vi "Termo_1.5__.vi"() -> ()   [LabVIEW 2015]
doc: "Программа мониторинга температуры"
panel:
  out "?":bool
  out "graph_update":bool
  out "Конфиг. АЦП?":bool
  in  "Tab Control":enum32{"ИЗМЕРЕНИЯ [К]", " АЦП", "ГРАФИК"}(tab)
  out "R2":dbl format="%.2f"
  in  "T2_visible":bool=TRUE
  in  "T5_visible":bool=TRUE
  out "R1":dbl format="%.2f"
  in  "T1_visible":bool=TRUE
  in  "T3_visible":bool=TRUE
  in  "T4_visible":bool=TRUE
  in  "T6_visible":bool=TRUE
  in  "stop":bool
  in  "ADC_dyn_range":T1(ring)=enum."± 0.625 В"
  in  "Buf_size":u8=1 min=1 max=128
  in  "SPS":T2(ring)
  in  "IP-адрес":string="192.168.127.254"
  in  "порт":u16=4001
  in  "Очистить график":bool
  in  "load_coeff.":bool caption="Disconn"
  in  "save_coeff.":bool caption="Disconn"
  in  "Coeff_cl_ch5":T3={"k1"=19.4736079181311652, "k2"=-232.79779903171584, "k3"=1229.13228608109057005, "k4"=-3103.0388431325554801, "k5"=4219.3520172238349901, "k6"=-2697.7160155214369299, "k7"=779.55193291697651198} caption="Канал 5" {"k7" format="%#_16g"; "k6" format="%#_16g"; "k5" format="%#_16g"; "k4" format="%#_16g"; "k3" format="%#_16g"; "k2" format="%#_16g"; "k1" format="%#_16g"}
  in  "Coeff_cl_ch4":T3={"k1"=24.218377729237545301, "k2"=-311.679773783311248, "k3"=1734.44359050504863, "k4"=-4665.87189712375402, "k5"=6719.3289510309696202, "k6"=-4578.02570509165525, "k7"=1400.00134176202118} caption="Канал 4" {"k7" format="%#_16g"; "k6" format="%#_16g"; "k5" format="%#_16g"; "k4" format="%#_16g"; "k3" format="%#_16g"; "k2" format="%#_16g"; "k1" format="%#_16g"}
  in  "Coeff_cl_ch3":T3={"k1"=8.756, "k2"=-142.210000000000000006, "k3"=1253.0, "k4"=-4877.1, "k5"=10581.0, "k6"=-10354.0, "k7"=3998.5} caption="Канал 3" {"k7" format="%#_16g"; "k6" format="%#_16g"; "k5" format="%#_16g"; "k4" format="%#_16g"; "k3" format="%#_16g"; "k2" format="%#_16g"; "k1" format="%#_16g"}
  in  "Coeff_cl_ch2":T3={"k1"=31.9101907935109921, "k2"=-399.867376562207937, "k3"=2119.32627579197288, "k4"=-5531.15447566658258, "k5"=7772.21873644739389, "k6"=-5292.23886113613844, "k7"=1613.2211984321475} caption="Канал 2" {"k7" format="%#_16g"; "k6" format="%#_16g"; "k5" format="%#_16g"; "k4" format="%#_16g"; "k3" format="%#_16g"; "k2" format="%#_16g"; "k1" format="%#_16g"}
  in  "Coeff_cl_ch6":T3={"k1"=11.9061392787261866, "k2"=-139.902402561856434, "k3"=774.882810204289854, "k4"=-1837.4832512177527, "k5"=2139.5822282396256899, "k6"=-730.555961686186492, "k7"=169.810834781266749} caption="Канал 6" {"k7" format="%#_16g"; "k6" format="%#_16g"; "k5" format="%#_16g"; "k4" format="%#_16g"; "k3" format="%#_16g"; "k2" format="%#_16g"; "k1" format="%#_16g"}
  in  "GraphLookB":bool
  in  "xScale -":bool
  in  "xScale +":bool
  out "мин.":string="1"
  in  "Старт измер.":bool
  in  "Стоп измер.":bool
  in  "Добавить время":dbl(ring)=300.0 items=["10 сек."=10.0, "1 мин."=60.0, "5 мин."=300.0, "20 мин."=1200.0]
  in  "min":dbl=4.0
  in  "max":dbl=300.0
  out "часы":string="0"
  in  "Autoscale":bool=TRUE
  out "сек.":string="0"
  out "Сутки":string
  out "счетчик":u32=4001
  in  "Запись в файл":bool
  in  "header?":bool caption="Disconn"
  out "con ID":refnum<k5>
  out "Graphs T":dynamicdata(graph) caption="U, мВ"
  # "U, мВ"
  # "Канал 1"
  # "Канал 2"
  # "Скорость измерений"
  # "SPS = Samples Per Second"
  # "Размер буфера усреднения"
  # "Диапазон измерений"
  # "Подключение"
  # "Шкала"
  # "Время графика"
  # ":"
  # ":"
  # "Измерения"
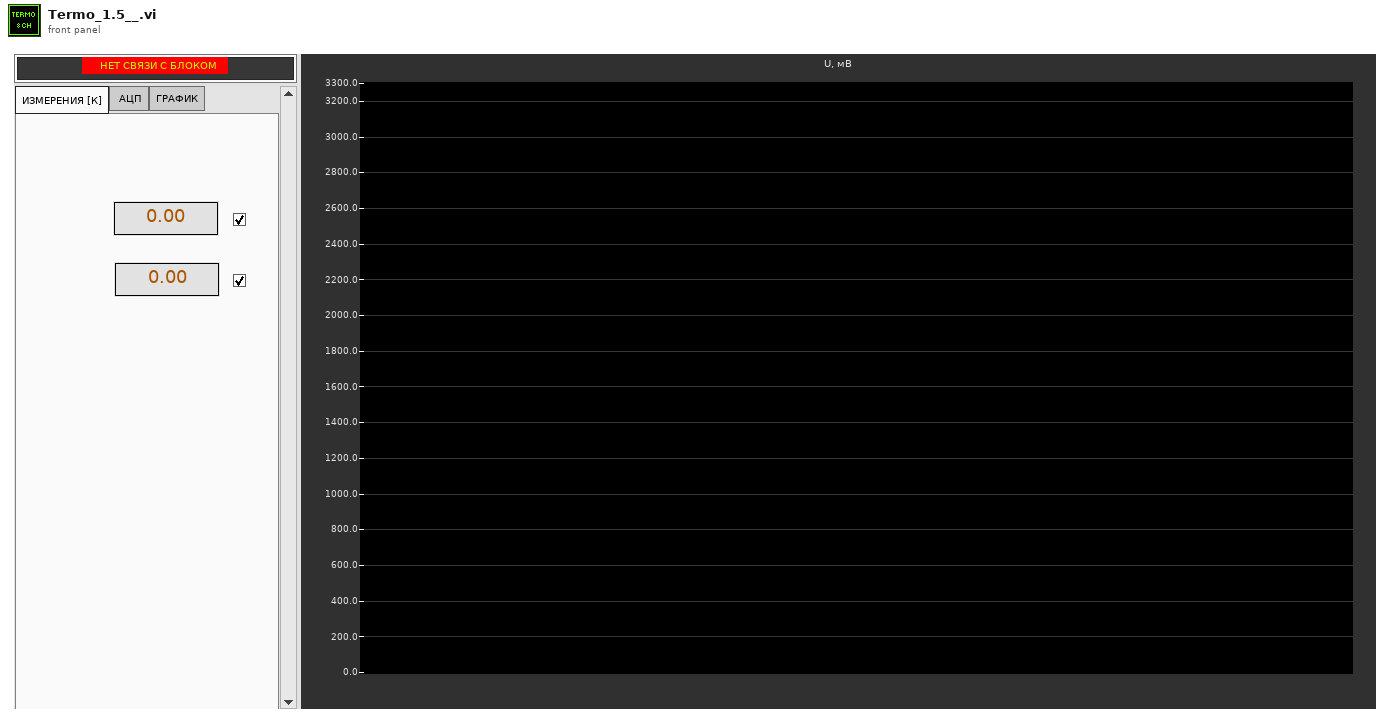
[diagram p1: front panel]
types:
  T1 = enum16{"± 5 В", "± 2.5 В", "± 1.25 В", "± 0.625 В", "± 312.5 мВ", "± 156.25 мВ", "± 78.125 мВ"}
  T2 = enum16{"2,5 SPS", "5 SPS", "10 SPS", "25 SPS", "50 SPS", "100 SPS", "500 SPS"}
  T3 = cluster{"k1":ext, "k2":ext, "k3":ext, "k4":ext, "k5":ext, "k6":ext, "k7":ext}
  T4 = enum32{"Page Enabled", "Page Disabled", "Page Disabled & Grayed"}
  T5 = enum16{"Standard", "Buffered", "CRLF", "Immediate"}
  T6 = typedef "LVDateTimeRec.ctl" = cluster{"fractional second":dbl, "second":i32, "minute":i32, "hour":i32, "day of month":i32, "month":i32, "year":i32, "day of week":i32, "day of year":i32, "DST":i32}
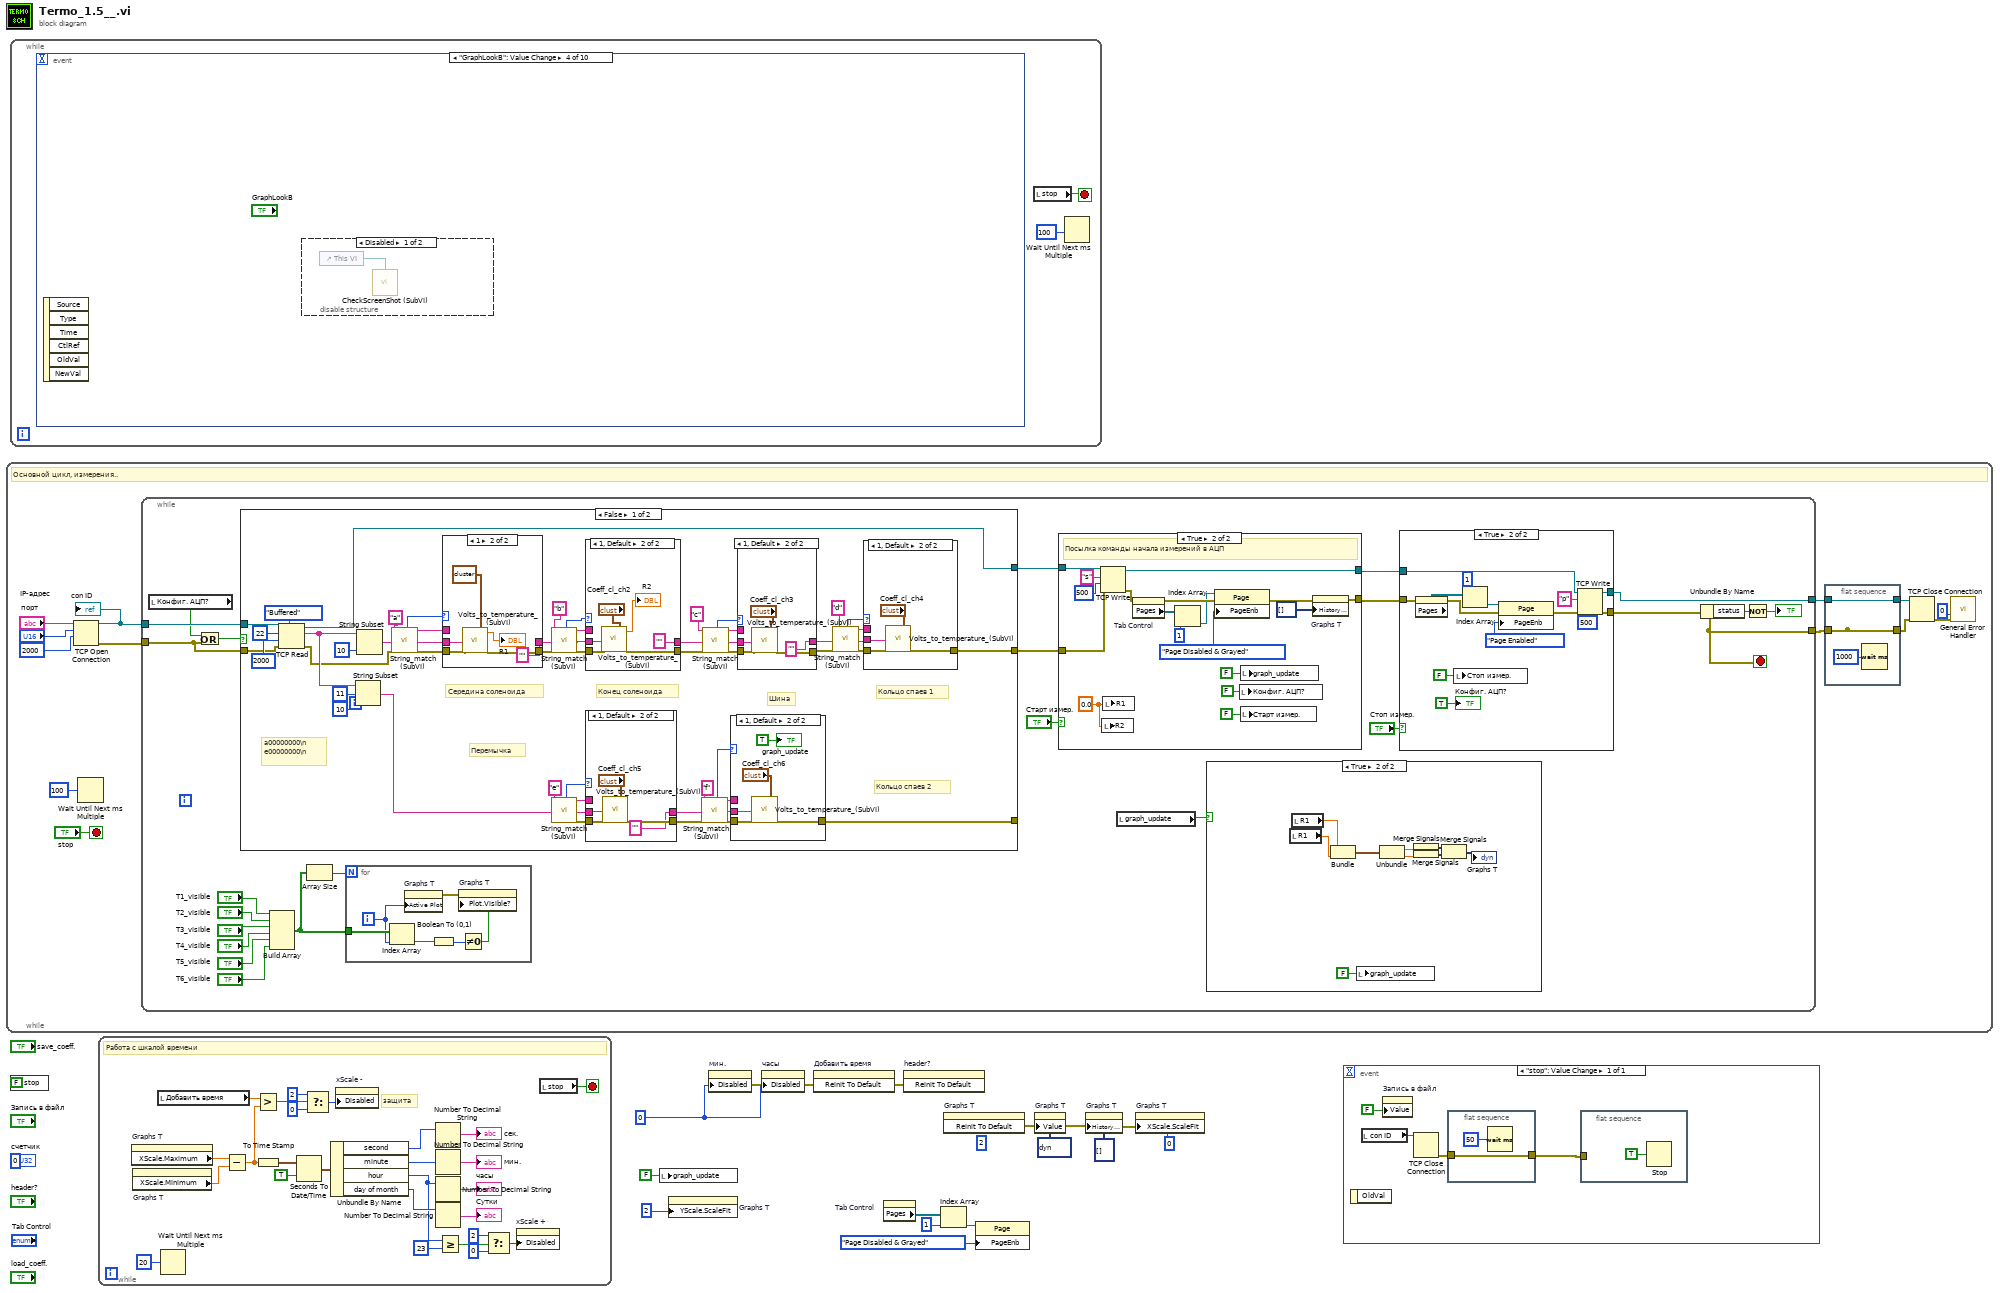
[diagram p0: block diagram]
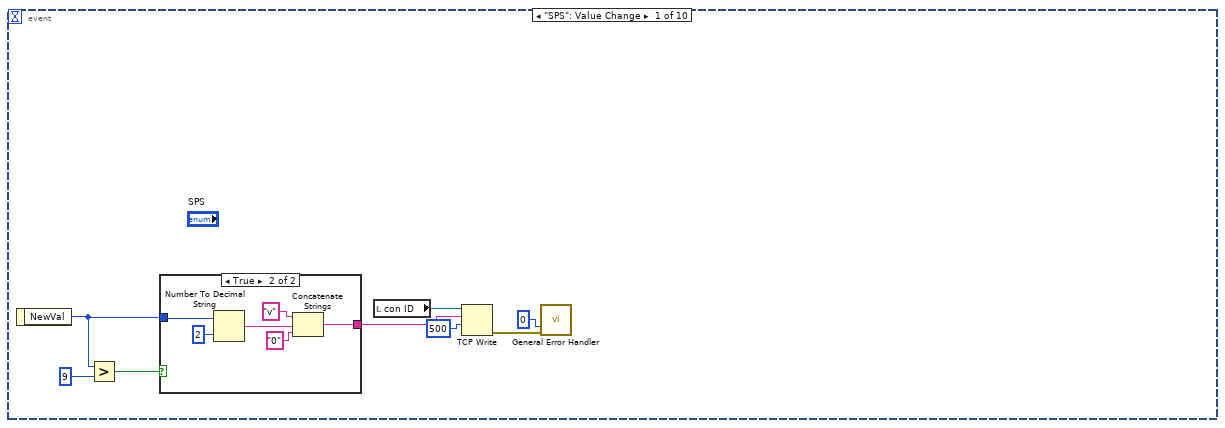
[diagram p2: hidden frame]
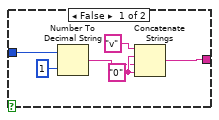
[diagram p3: hidden frame]
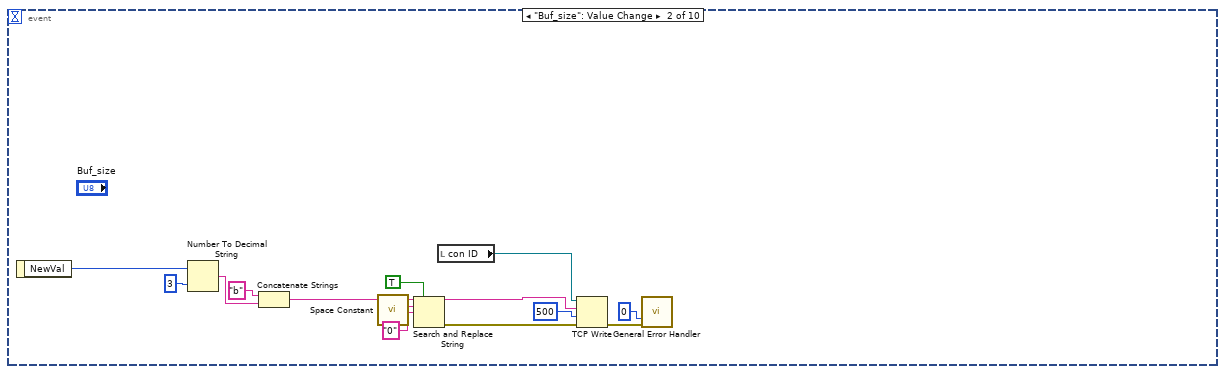
[diagram p4: hidden frame]
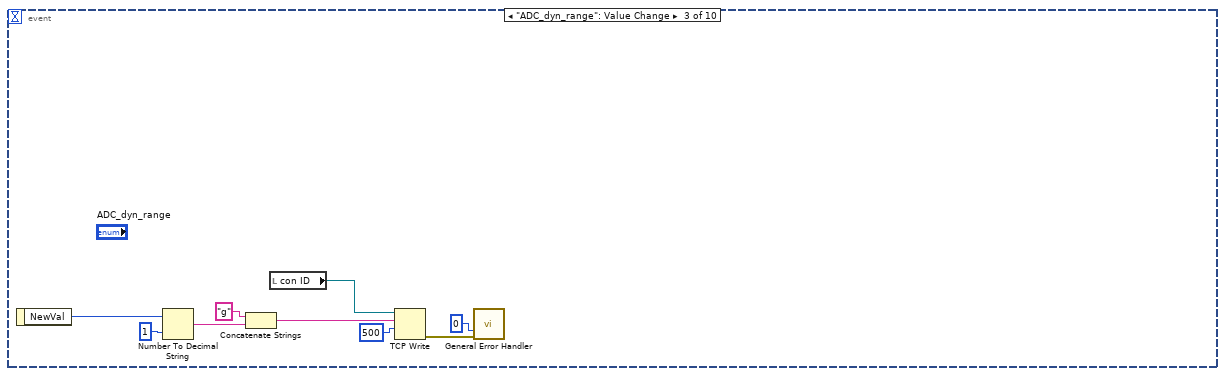
[diagram p5: hidden frame]
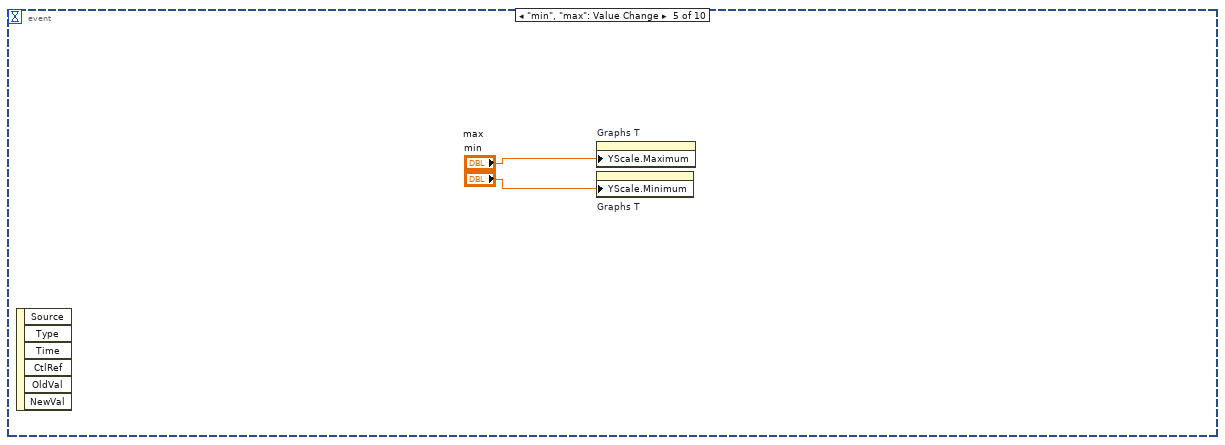
[diagram p7: hidden frame]
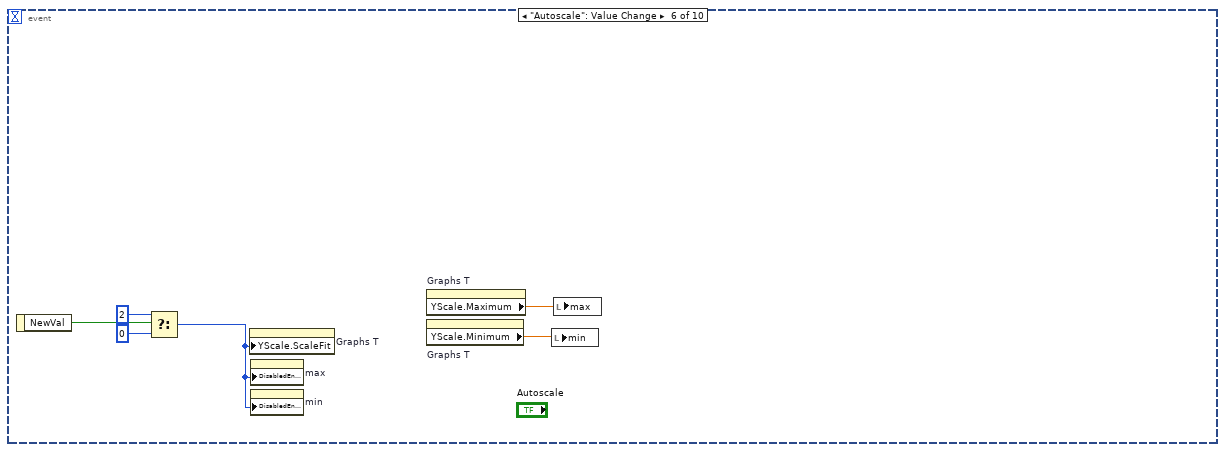
[diagram p8: hidden frame]
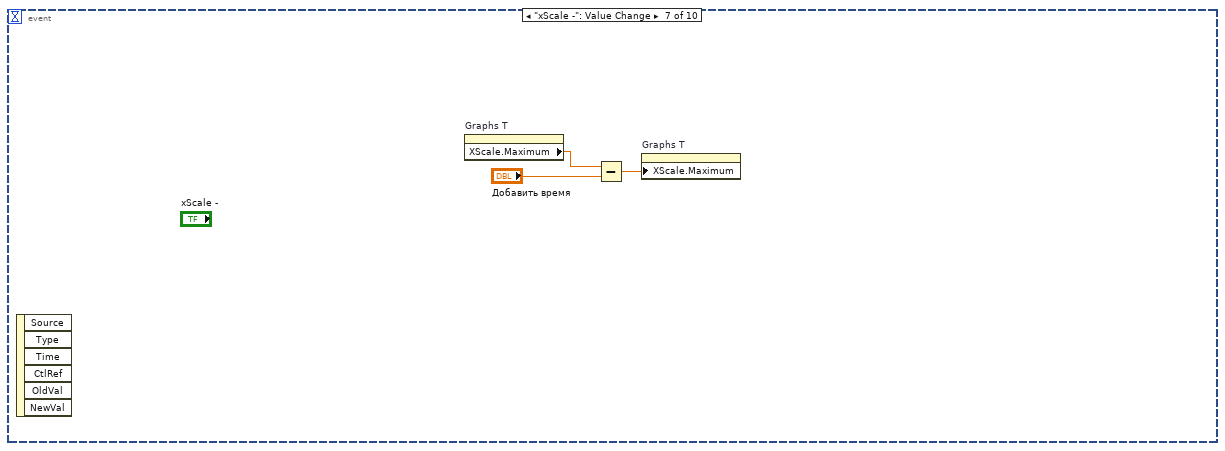
[diagram p9: hidden frame]
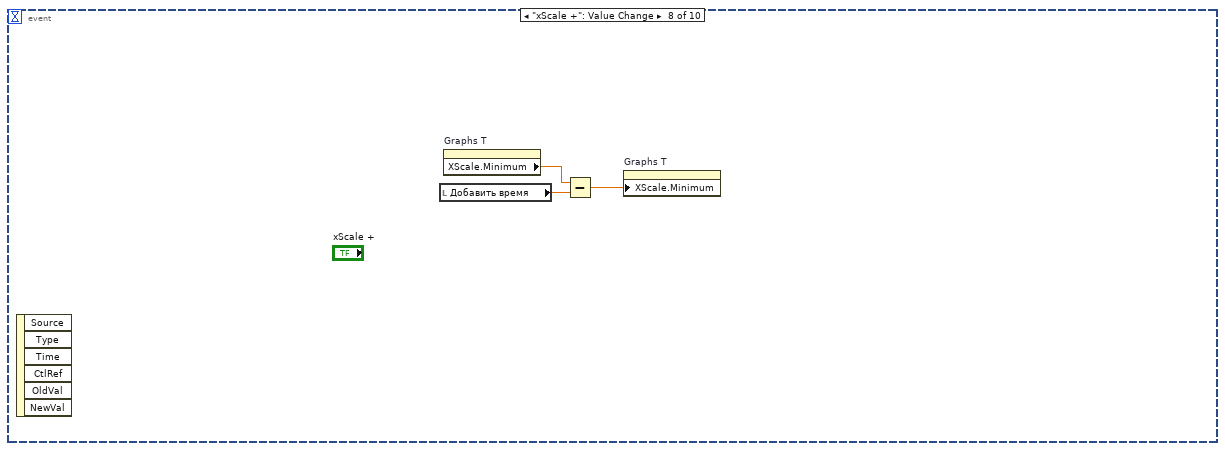
[diagram p10: hidden frame]
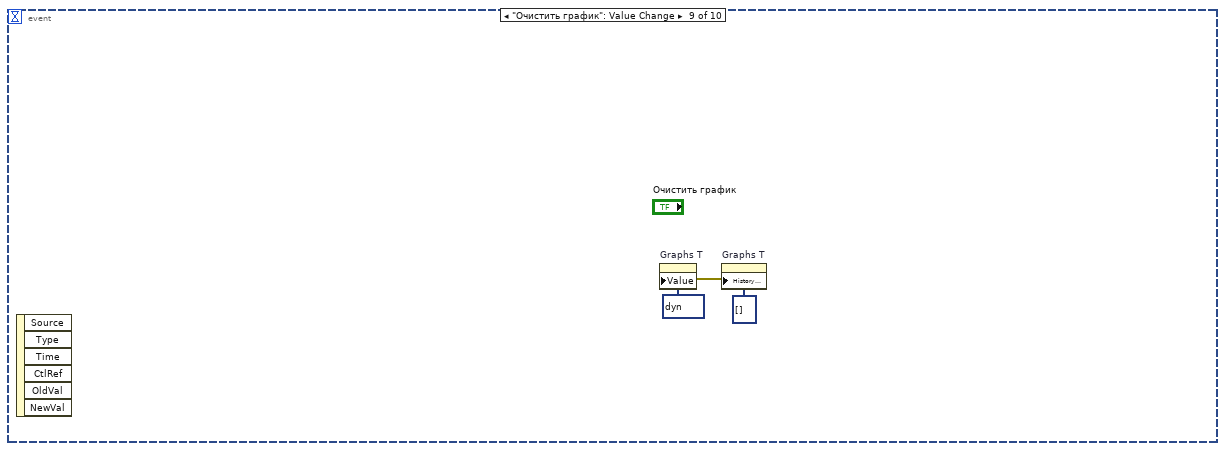
[diagram p11: hidden frame]
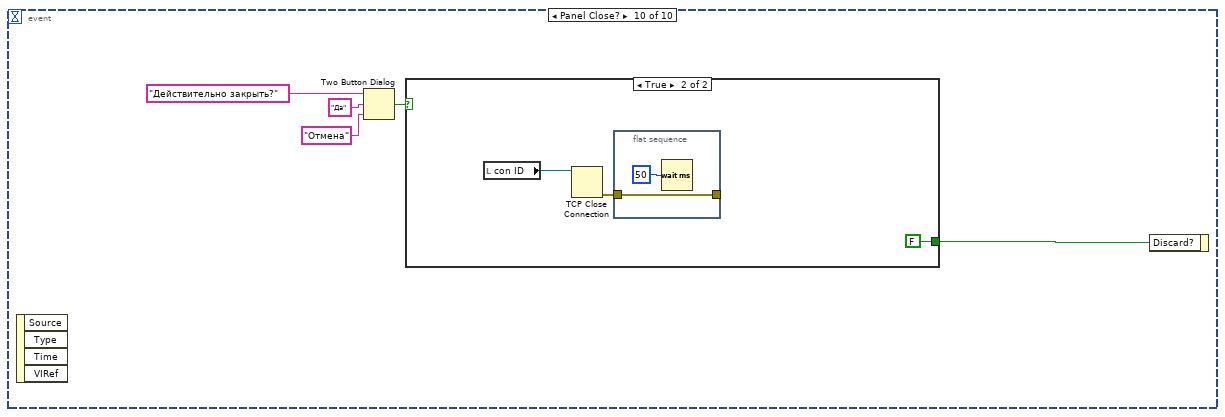
[diagram p12: hidden frame]
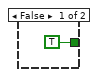
[diagram p13: hidden frame]
diagram:
  w18 = u8 0 ("Disabled")
  (unwired) u8 2 ("Disabled")
  n1 = while {
    stop <- "stop" stop-if-true
    # "Основной цикл, измерения.."
    n2 = TCP Open Connection(address="IP-адрес", remote port or service name="порт", timeout ms (60000)=2000) -> (connection ID=w30:refnum<k5>, error out=w24:errorcluster)  [unwired: 1 in, 1 out]
    "con ID" <- w30
    n3 = Wait Until Next ms Multiple(millisecond multiple=u32 100) -> ()  [unwired: 1 out]
    n4 = while {
      tunnel: w30 -> [w57]
      tunnel: w24 -> [w40]
      tunnel: [w36] -> w22
      tunnel: [w35] -> w20
      stop <- w35 stop-if-true
      n5 = local read "Конфиг. АЦП?"() -> (w41:bool)
      n6 = Or(x=w41, y=w40) -> (x .or. y?=w55:bool)
      n7 = case shown="False" w55 {
        tunnel: [w111 w204] -> w42
        tunnel: w57 -> [w114 w204]
        tunnel: [w110 w203] -> w38
        tunnel: w40 -> [w112 w203]
        tunnel: [w109 _] -> _
        frame False {
          # "a00000000\\n\ne00000000\\n"
          # "Кольцо спаев 2"
          # "Шина"
          # "Перемычка"
          # "Кольцо спаев 1"
          # "Конец соленоида"
          # "Середина соленоида"
          n8 = TCP Read(connection ID=w114, bytes to read=22, error in (no error)=w112, 7:T5."Buffered" ("mode (standard)"), 9:2000 ("timeout ms (25000)")) -> (connection ID out=w111:refnum<k5>, data out=w118:string, error out=w113:errorcluster)
          n9 = String Subset(string=w118, offset (0)=11, length (rest)=10 ("length (rest)")) -> (substring=w115:string)
          n10 = String Subset(string=w118, length (rest)=10 ("length (rest)")) -> (substring=w120:string)  [unwired: 1 in]
          n11 = call "String_match (SubVI).vi"("channel id"="a" ("regular expression"), "input string"=w120, "error in"=w113) -> ("match ?"=w126:i32, "output string"=w154:string, "match substring"=w155:string, "error out"=w156:errorcluster)  [unwired: 13 in]
          n12 = case shown="1" w126 {
            tunnel: [w196 w201] -> w145
            tunnel: w156 -> [w196 w202]
            tunnel: w155 -> [_ w198]
            tunnel: [w195 "" ("output string")] -> w158
            tunnel: w154 -> [w195 _]
            frame -1, Default {
            }
            frame 1 {
              n13 = call "Volts_to_temperature_(SubVI).vi"("ch_data_string"=w198, "error in"=w202, "koeff. cluster"=T3 {"k1"=20.678416953771299999, "k2"=-270.806564304511, "k3"=1559.71508308313, "k4"=-4317.07993103563, "k5"=6444.9990497231400002, "k6"=-4562.30018320679, "k7"=1455.99202726967}) -> ("meas_voltage mV"=→"R1":dbl, "error out"=w201:errorcluster)  [unwired: 20 in, 3 out]
            }
          }
          n14 = call "String_match (SubVI).vi"("channel id"="b" ("regular expression"), "input string"=w158, "error in"=w145) -> ("match ?"=w125:i32, "output string"=w150:string, "match substring"=w151:string, "error out"=w152:errorcluster)  [unwired: 13 in]
          n15 = call "String_match (SubVI).vi"("channel id"="e" ("regular expression"), "input string"=w115) -> ("match ?"=w122:i32, "output string"=w143:string, "match substring"=w142:string, "error out"=w141:errorcluster)  [unwired: 14 in]
          n16 = case shown="1, Default" w125 {
            tunnel: [w188 w194] -> w134
            tunnel: w152 -> [w188 w193]
            tunnel: w151 -> [_ w192]
            tunnel: w150 -> [w187 _]
            tunnel: [w187 "" ("output string")] -> w133
            frame -1 {
            }
            frame 1, Default {
              n17 = call "Volts_to_temperature_(SubVI).vi"("ch_data_string"=w192, "error in"=w193, "koeff. cluster"="Coeff_cl_ch2") -> ("meas_voltage mV"=→"R2":dbl, "error out"=w194:errorcluster)  [unwired: 20 in, 3 out]
            }
          }
          n18 = case shown="1, Default" w122 {
            tunnel: [w176 w181] -> w144
            tunnel: w141 -> [w176 w180]
            tunnel: w142 -> [_ w179]
            tunnel: [w175 "" ("output string")] -> w139
            tunnel: w143 -> [w175 _]
            frame -1 {
            }
            frame 1, Default {
              n19 = call "Volts_to_temperature_(SubVI).vi"("ch_data_string"=w179, "error in"=w180, "koeff. cluster"="Coeff_cl_ch5") -> ("error out"=w181:errorcluster)  [unwired: 20 in, 4 out]
            }
          }
          n20 = call "String_match (SubVI).vi"("channel id"="f" ("regular expression"), "input string"=w139, "error in"=w144) -> ("match ?"=w121:i32, "output string"=w138:string, "match substring"=w137:string, "error out"=w136:errorcluster)  [unwired: 13 in]
          n21 = call "String_match (SubVI).vi"("channel id"="c" ("regular expression"), "input string"=w133, "error in"=w134) -> ("match ?"=w124:i32, "output string"=w129:string, "match substring"=w130:string, "error out"=w131:errorcluster)  [unwired: 13 in]
          n22 = case shown="1, Default" w121 {
            tunnel: [w169 w174] -> w109
            tunnel: w136 -> [w169 w173]
            tunnel: w137 -> [_ w172]
            tunnel: w138 -> [_ _]
            frame -1 {
            }
            frame 1, Default {
              n23 = call "Volts_to_temperature_(SubVI).vi"("ch_data_string"=w172, "error in"=w173, "koeff. cluster"="Coeff_cl_ch6") -> ("error out"=w174:errorcluster)  [unwired: 20 in, 4 out]
              "graph_update" <- TRUE ("graph_update")
            }
          }
          n24 = case shown="1, Default" w124 {
            tunnel: w131 -> [w163 w167]
            tunnel: [w163 w166] -> w128
            tunnel: w130 -> [_ w165]
            tunnel: w129 -> [w162 _]
            tunnel: [w162 "" ("output string")] -> w127
            frame -1 {
            }
            frame 1, Default {
              n25 = call "Volts_to_temperature_(SubVI).vi"("ch_data_string"=w165, "error in"=w167, "koeff. cluster"="Coeff_cl_ch3") -> ("error out"=w166:errorcluster)  [unwired: 20 in, 4 out]
            }
          }
          n26 = call "String_match (SubVI).vi"("channel id"="d" ("regular expression"), "input string"=w127, "error in"=w128) -> ("match ?"=w123:i32, "output string"=w146:string, "match substring"=w147:string, "error out"=w148:errorcluster)  [unwired: 13 in]
          n27 = case shown="1, Default" w123 {
            tunnel: w148 -> [w182 w186]
            tunnel: [w182 w185] -> w110
            tunnel: w147 -> [_ w184]
            tunnel: w146 -> [_ _]
            frame -1 {
            }
            frame 1, Default {
              n28 = call "Volts_to_temperature_(SubVI).vi"("ch_data_string"=w184, "error in"=w186, "koeff. cluster"="Coeff_cl_ch4") -> ("error out"=w185:errorcluster)  [unwired: 20 in, 4 out]
            }
          }
        }
        frame True {
        }
      }
      n29 = Build Array("T1_visible", "T2_visible", "T3_visible", "T4_visible", "T5_visible", "T6_visible") -> (w47:bool[])
      n30 = Array Size(array=w47) -> (size(s)=w48:i32)
      n31 = for {
        N: w48 -> [_]
        tunnel: w47 -> [w107]
        i -> [w105]
        n32 = Index Array(array=w107, index=w105) -> (element=w104:bool)
        n33 = property on="Graphs T" class="WFChart (strict)"("Active Plot"=w105) -> (error out=w106:errorcluster)  [unwired: 2 in, 1 out]
        n34 = Boolean To (0,1)(Boolean=w104) -> (0, 1=w108:i16)
        n35 = Not Equal To 0?(x=w108) -> (x != 0?=w103:bool)
        n36 = property on="Graphs T" class="WFChart (strict)"(error in=w106, "Plot.Visible?"=w103) -> ()  [unwired: 1 in, 2 out]
      }
      n37 = case shown="True" "Старт измер." {
        tunnel: [w83 w92] -> w44
        tunnel: [w84 w91] -> w46
        tunnel: w42 -> [w84 w88]
        tunnel: w38 -> [w83 w87]
        frame False {
        }
        frame True {
          w85 = 0.0 ("3")
          # "Посылка команды начала измерений в АЦП"
          n38 = TCP Write(connection ID=w88, data in="s", error in (no error)=w87, 9:500 ("timeout ms (25000)")) -> (connection ID out=w91:refnum<k5>, error out=w100:errorcluster)  [unwired: 1 out]
          n39 = local write "R2"(w85) -> ()
          n40 = local write "R1"(w85) -> ()
          n41 = property on="Tab Control" class="TabCtl (strict)"(error in=w100) -> (error out=w101:errorcluster, "Pages"=w96:refnum<vi>[])  [unwired: 1 in, 1 out]
          n42 = Index Array(array=w96, index=1) -> (element=w97:refnum<vi>)
          n43 = property class="Page"(reference=w97, error in=w101, "PageEnb"=T4."Page Disabled & Grayed" ("Page Enabled State")) -> (error out=w89:errorcluster)  [unwired: 1 out]
          n44 = local write "Конфиг. АЦП?"(FALSE ("Старт измер.")) -> ()
          n45 = local write "graph_update"(FALSE ("graph_update")) -> ()
          n46 = local write "Старт измер."(FALSE ("Старт измер.")) -> ()
          n47 = property on="Graphs T" class="WFChart (strict)"(error in=w89, "History Data"=dynamicdata[] []) -> (error out=w92:errorcluster)  [unwired: 1 in, 1 out]
        }
      }
      n48 = local read "graph_update"() -> (w37:bool)
      n49 = case shown="True" w37 {
        frame False {
        }
        frame True {
          n50 = local read "R1"() -> (w64:dbl)
          n51 = local read "R1"() -> (w65:dbl)
          n52 = Bundle("R1"=w65, "R1"=w64) -> (w63:cluster{" R1":dbl, " R1":dbl})  [unwired: 1 in]
          n53 = local write "graph_update"(FALSE ("graph_update")) -> ()
          n54 = Unbundle(w63) -> ("R1"=w59:dbl, "R1"=w58:dbl)
          n55 = Merge Signals(w59) -> (w61:dynamicdata)
          n56 = Merge Signals(w58) -> (w62:dynamicdata)
          n57 = Merge Signals(w61, w62) -> (→"Graphs T":dynamicdata)
        }
      }
      n58 = case shown="True" "Стоп измер." {
        tunnel: w44 -> [w67 w75]
        tunnel: w46 -> [w68 w73]
        tunnel: [w67 w69] -> w35
        tunnel: [w68 w70] -> w36
        frame False {
        }
        frame True {
          n59 = property on="Tab Control" class="TabCtl (strict)"(error in=w75) -> (error out=w74:errorcluster, "Pages"=w78:refnum<vi>[])  [unwired: 1 in, 1 out]
          n60 = local write "Стоп измер."(FALSE ("Стоп измер.")) -> ()
          n61 = Index Array(array=w78, index=1) -> (element=w79:refnum<vi>)
          n62 = property class="Page"(reference=w79, error in=w74, "PageEnb"=T4."Page Enabled" ("Page Enabled State")) -> (error out=w82:errorcluster)  [unwired: 1 out]
          n63 = TCP Write(connection ID=w73, data in="p", error in (no error)=w82, 9:500 ("timeout ms (25000)")) -> (connection ID out=w70:refnum<k5>, error out=w69:errorcluster)  [unwired: 1 out]
          "Конфиг. АЦП?" <- TRUE ("Конфиг. АЦП?")
        }
      }
      n64 = Unbundle By Name(w35) -> ("status"=w39:bool)
      n65 = Not(x=w39) -> (.not. x?=→"?":bool)
    }
    n66 = flat-sequence {
      tunnel: [w33] -> w21
      tunnel: w22 -> [w33]
      tunnel: w20 -> [w32]
      tunnel: [w32] -> _
      tunnel: [w32] -> w19
      frame #0 {
        n67 = Wait (ms)(milliseconds to wait=u32 1000) -> ()  [unwired: 1 out]
      }
    }
    n68 = TCP Close Connection(connection ID=w21, error in (no error)=w19) -> (error out=w29:errorcluster)  [unwired: 2 out]
    n69 = call <vilib>:"General Error Handler.vi"("type of dialog (OK msg:1)"=u32 0 ("milliseconds to wait"), "error in (no error)"=w29) -> ()  [unwired: 1 in, 13 out]
  }
  n70 = while {
    stop <- w205 stop-if-true
    n71 = event shown="[3] \"GraphLookB\": Value Change" {
      selector: _ -> [_ _ _ _ _ _ _ _ _ _]
      dyn-events: _ -> [_ _ _ _ _ _ _ _ _ _]
      timeout: _ -> [_ _ _ _ _ _ _ _ _ _]
      event "SPS": Value Change {
        n72 = event-data() -> ("NewVal"=w210:T2)  [unwired: 1 in]
        n73 = Greater?(x=w210, y=9 ("timeout ms (25000)")) -> (0:w208:bool)
        n74 = case shown="True" w208 {
          tunnel: w210 -> [w220 w226]
          tunnel: [w217 w221] -> w207
          frame False {
            w216 = "0" ("string")
            n75 = Number To Decimal String(number=w220, width (-)=i16 1) -> (decimal integer string=w215:string)
            n76 = Concatenate Strings("v" ("data in"), w216, w215, w216) -> (w217:string)
          }
          frame True {
            n77 = Number To Decimal String(number=w226, width (-)=i16 2) -> (decimal integer string=w223:string)
            n78 = Concatenate Strings("v" ("data in"), w223, "0" ("string")) -> (w221:string)
          }
        }
        n79 = local read "con ID"() -> (w213:refnum<k5>)
        n80 = TCP Write(connection ID=w213, data in=w207, 9:500 ("timeout ms (25000)")) -> (error out=w212:errorcluster)  [unwired: 1 in, 2 out]
        n81 = call <vilib>:"General Error Handler.vi"("type of dialog (OK msg:1)"=0 ("timeout ms (25000)"), "error in (no error)"=w212) -> ()  [unwired: 9 in, 5 out]
      }
      event "Buf_size": Value Change {
        n82 = event-data() -> ("NewVal"=w237:u8)  [unwired: 1 in]
        n83 = Number To Decimal String(number=w237, width (-)=i16 3) -> (decimal integer string=w235:string)
        n84 = Concatenate Strings("b" ("data in"), w235) -> (w234:string)
        n85 = call <vilib>:"Space Constant.vi"() -> ("String"=w232:string)
        n86 = Search and Replace String(replace all?=TRUE ("replace all? (F)"), input string=w234, search string=w232, replace string="0" ("replace string (\"\")")) -> (result string=w233:string, error out=w229:errorcluster)  [unwired: 4 in, 2 out]
        n87 = local read "con ID"() -> (w239:refnum<k5>)
        n88 = TCP Write(connection ID=w239, data in=w233, error in (no error)=w229, 9:500 ("timeout ms (25000)")) -> (error out=w228:errorcluster)  [unwired: 2 out]
        n89 = call <vilib>:"General Error Handler.vi"("type of dialog (OK msg:1)"=0 ("timeout ms (25000)"), "error in (no error)"=w228) -> ()  [unwired: 9 in, 5 out]
      }
      event "ADC_dyn_range": Value Change {
        n90 = event-data() -> ("NewVal"=w246:T1)  [unwired: 1 in]
        n91 = Number To Decimal String(number=w246, width (-)=i16 1) -> (decimal integer string=w244:string)
        n92 = Concatenate Strings("g" ("data in"), w244) -> (w243:string)
        n93 = local read "con ID"() -> (w248:refnum<k5>)
        n94 = TCP Write(connection ID=w248, data in=w243, 9:500 ("timeout ms (25000)")) -> (error out=w241:errorcluster)  [unwired: 1 in, 2 out]
        n95 = call <vilib>:"General Error Handler.vi"("type of dialog (OK msg:1)"=0 ("timeout ms (25000)"), "error in (no error)"=w241) -> ()  [unwired: 9 in, 5 out]
      }
      event "GraphLookB": Value Change {
        n96 = event-data() -> ()  [unwired: 1 in, 6 out]
        n97 = disable-structure shown="Disabled" {
          frame Disabled {
            n98 = control-ref of="This VI"() -> (w250:refnum<vi>)
            n99 = call "CheckScreenShot (SubVI).vi"("VI reference"=w250) -> ()  [unwired: 15 in]
          }
          frame Enabled {
          }
        }
      }
      event "min", "max": Value Change {
        n100 = event-data() -> ()  [unwired: 1 in, 6 out]
        n101 = property on="Graphs T" class="WFChart (strict)"("YScale.Maximum"="max") -> ()  [unwired: 2 in, 2 out]
        n102 = property on="Graphs T" class="WFChart (strict)"("YScale.Minimum"="min") -> ()  [unwired: 2 in, 2 out]
      }
      event "Autoscale": Value Change {
        n103 = event-data() -> ("NewVal"=w253:bool)  [unwired: 1 in]
        n104 = Select(t=u8 2 ("Y Scale.Scale Fit"), s=w253, f=u8 0 ("Y Scale.Scale Fit")) -> (s? t:f=w256:u8)
        n105 = property on="Graphs T" class="WFChart (strict)"("YScale.ScaleFit"=w256) -> ()  [unwired: 2 in, 2 out]
        n106 = property on="max" class="DigNum (strict)"("DisabledEnum"=w256) -> ()  [unwired: 2 in, 2 out]
        n107 = property on="min" class="DigNum (strict)"("DisabledEnum"=w256) -> ()  [unwired: 2 in, 2 out]
        n108 = property on="Graphs T" class="WFChart (strict)"() -> ("YScale.Maximum"=w254:dbl)  [unwired: 2 in, 2 out]
        n109 = property on="Graphs T" class="WFChart (strict)"() -> ("YScale.Minimum"=w255:dbl)  [unwired: 2 in, 2 out]
        n110 = local write "min"(w255) -> ()
        n111 = local write "max"(w254) -> ()
      }
      event "xScale -": Value Change {
        n112 = event-data() -> ()  [unwired: 1 in, 6 out]
        n113 = property on="Graphs T" class="WFChart (strict)"() -> ("XScale.Maximum"=w261:dbl)  [unwired: 2 in, 2 out]
        n114 = Subtract(x=w261, y="Добавить время") -> (x-y=w260:dbl)
        n115 = property on="Graphs T" class="WFChart (strict)"("XScale.Maximum"=w260) -> ()  [unwired: 2 in, 2 out]
      }
      event "xScale +": Value Change {
        n116 = event-data() -> ()  [unwired: 1 in, 6 out]
        n117 = local read "Добавить время"() -> (w262:dbl)
        n118 = property on="Graphs T" class="WFChart (strict)"() -> ("XScale.Minimum"=w264:dbl)  [unwired: 2 in, 2 out]
        n119 = Subtract(x=w264, y=w262) -> (x-y=w263:dbl)
        n120 = property on="Graphs T" class="WFChart (strict)"("XScale.Minimum"=w263) -> ()  [unwired: 2 in, 2 out]
      }
      event "Очистить график": Value Change {
        n121 = event-data() -> ()  [unwired: 1 in, 6 out]
        n122 = property on="Graphs T" class="WFChart (strict)"("Value"=dynamicdata [{"t0"=timestamp(3465273261.7246556 s since 1904-01-01), "dt"=1.0, "Y"=[0.1931097262457384]}, {"t0"=timestamp(3465273261.7246556 s since 1904-01-01), "dt"=1.0, "Y"=[0.3594116459482981]}, {"t0"=timestamp(3465273261.7246556 s since 1904-01-01), "dt"=1.0, "Y"=[0.8898205452798131]}, {"t0"=timestamp(3465273261.7246556 s since 1904-01-01), "dt"=1.0, "Y"=[0.747699236883661]}] ("Graphs")) -> (error out=w266:errorcluster)  [unwired: 2 in, 1 out]
        n123 = property on="Graphs T" class="WFChart (strict)"(error in=w266, "History Data"=dynamicdata[] []) -> ()  [unwired: 1 in, 2 out]
      }
      event Panel Close? {
        n124 = event-data() -> ()  [unwired: 1 in, 4 out]
        n125 = Two Button Dialog(message="Действительно закрыть?", 1:"Отмена" ("T button name (\"OK\")"), 2:"Да" ("T button name (\"OK\")")) -> (T button?=w269:bool)
        n126 = case shown="True" w269 {
          tunnel: [TRUE ("Discard?") FALSE ("Discard?")] -> w268
          frame False {
          }
          frame True {
            n127 = local read "con ID"() -> (w275:refnum<k5>)
            n128 = TCP Close Connection(connection ID=w275) -> (error out=w276:errorcluster)  [unwired: 1 in, 2 out]
            n129 = flat-sequence {
              tunnel: [w277] -> _
              tunnel: w276 -> [w277]
              frame #0 {
                n130 = Wait (ms)(milliseconds to wait=u32 50) -> ()  [unwired: 1 out]
              }
            }
          }
        }
        n131 = event-data("Discard?"=w268) -> ()  [unwired: 1 in, 1 out]
      }
    }
    n132 = local read "stop"() -> (w205:bool)
    n133 = Wait Until Next ms Multiple(millisecond multiple=u32 100 ("milliseconds to wait")) -> ()  [unwired: 1 out]
  }
  n134 = local write "stop"(FALSE ("Boolean")) -> ()
  n135 = while {
    stop <- w304 stop-if-true
    # "защита"
    # "Работа с шкалой времени"
    n136 = property on="Graphs T" class="WFChart (strict)"() -> ("XScale.Maximum"=w280:dbl)  [unwired: 2 in, 2 out]
    n137 = property on="Graphs T" class="WFChart (strict)"() -> ("XScale.Minimum"=w279:dbl)  [unwired: 2 in, 2 out]
    n138 = local read "Добавить время"() -> (w303:dbl)
    n139 = Wait Until Next ms Multiple(millisecond multiple=u32 20) -> ()  [unwired: 1 out]
    n140 = Subtract(x=w280, y=w279) -> (x-y=w293:dbl)
    n141 = Greater?(x=w303, y=w293) -> (0:w286:bool)
    n142 = To Time Stamp(1:w293) -> (0:w301:timestamp)
    n143 = Seconds To Date/Time(time stamp (now)=w301, to UTC (F)=TRUE) -> (date time rec=w300:T6)
    n144 = Select(t=u8 2 ("Disabled"), s=w286, f=u8 0 ("Disabled")) -> (s? t:f=w289:u8)
    n145 = Unbundle By Name(w300) -> ("second"=w299:i32, "minute"=w298:i32, "hour"=w291:i32, "day of month"=w297:i32)
    n146 = property on="xScale -" class="Bool (strict)"("Disabled"=w289) -> ()  [unwired: 2 in, 2 out]
    n147 = Number To Decimal String(number=w299) -> (decimal integer string=→"сек.":string)  [unwired: 1 out]
    n148 = Number To Decimal String(number=w298) -> (decimal integer string=→"мин.":string)  [unwired: 1 out]
    n149 = Number To Decimal String(number=w291) -> (decimal integer string=→"часы":string)  [unwired: 1 out]
    n150 = Number To Decimal String(number=w297) -> (decimal integer string=→"Сутки":string)  [unwired: 1 out]
    n151 = Greater Or Equal?(x=w291, y=23) -> (x >= y?=w282:bool)
    n152 = Select(t=u8 2 ("Disabled"), s=w282, f=u8 0 ("Disabled")) -> (s? t:f=w285:u8)
    n153 = property on="xScale +" class="Bool (strict)"("Disabled"=w285) -> ()  [unwired: 2 in, 2 out]
    n154 = local read "stop"() -> (w304:bool)
  }
  n155 = local write "graph_update"(FALSE ("graph_update")) -> ()
  n156 = property on="Graphs T" class="WFChart (strict)"("YScale.ScaleFit"=u8 2 ("Y Scale.Scale Fit")) -> ()  [unwired: 2 in, 2 out]
  n157 = property on="мин." class="Str"("Disabled"=w18) -> (error out=w17:errorcluster)  [unwired: 2 in, 1 out]
  n158 = property on="часы" class="Str"(error in=w17, "Disabled"=w18) -> (error out=w16:errorcluster)  [unwired: 1 in, 1 out]
  n159 = invoke on="Добавить время" class="Ring (strict)" method="Reinit To Default"(error in=w16) -> (error out=w11:errorcluster)  [unwired: 2 in, 2 out]
  n160 = property on="Tab Control" class="TabCtl (strict)"() -> ("Pages"=w12:refnum<vi>[])  [unwired: 2 in, 2 out]
  n161 = invoke on="header?" class="Bool (strict)" method="Reinit To Default"(error in=w11) -> ()  [unwired: 2 in, 3 out]
  n162 = Index Array(array=w12, index=1) -> (element=w13:refnum<vi>)
  n163 = invoke on="Graphs T" class="WFChart (strict)" method="Reinit To Default"() -> (error out=w7:errorcluster)  [unwired: 3 in, 2 out]
  n164 = property class="Page"(reference=w13, "PageEnb"=T4."Page Disabled & Grayed" ("Page Enabled State")) -> ()  [unwired: 1 in, 2 out]
  n165 = property on="Graphs T" class="WFChart (strict)"(error in=w7, "Value"=dynamicdata [{"t0"=timestamp(3465273261.7246556 s since 1904-01-01), "dt"=1.0, "Y"=[0.1931097262457384]}, {"t0"=timestamp(3465273261.7246556 s since 1904-01-01), "dt"=1.0, "Y"=[0.3594116459482981]}, {"t0"=timestamp(3465273261.7246556 s since 1904-01-01), "dt"=1.0, "Y"=[0.8898205452798131]}, {"t0"=timestamp(3465273261.7246556 s since 1904-01-01), "dt"=1.0, "Y"=[0.747699236883661]}] ("Graphs")) -> (error out=w6:errorcluster)  [unwired: 1 in, 1 out]
  n166 = property on="Graphs T" class="WFChart (strict)"(error in=w6, "History Data"=dynamicdata[] []) -> (error out=w10:errorcluster)  [unwired: 1 in, 1 out]
  n167 = property on="Graphs T" class="WFChart (strict)"(error in=w10, "XScale.ScaleFit"=u8 0 ("Y Scale.Scale Fit")) -> ()  [unwired: 1 in, 2 out]
  n168 = event shown="[0] \"stop\": Value Change" {
    selector: _ -> [_]
    dyn-events: _ -> [_]
    timeout: _ -> [_]
    event "stop": Value Change {
      n169 = event-data() -> ()  [unwired: 1 in, 1 out]
      n170 = local read "con ID"() -> (w306:refnum<k5>)
      n171 = property on="Запись в файл" class="Bool (strict)"("Value"=FALSE ("Запись в файл")) -> ()  [unwired: 2 in, 2 out]
      n172 = TCP Close Connection(connection ID=w306) -> (error out=w308:errorcluster)  [unwired: 1 in, 2 out]
      n173 = flat-sequence {
        tunnel: [w310] -> w305
        tunnel: w308 -> [w310]
        frame #0 {
          n174 = Wait (ms)(milliseconds to wait=u32 50) -> ()  [unwired: 1 out]
        }
      }
      n175 = flat-sequence {
        tunnel: w305 -> [_]
        frame #0 {
          n176 = Stop(stop? (T)=TRUE) -> ()
        }
      }
    }
  }
  "счетчик" <- u32 0 ("счетчик")
